vi "Create.vi"(5 "TestFailure In":refnum<class "TestFailure.lvclass">, 8 "error in (no error)":errorcluster, 9 "Failure":errorcluster, 10 "Test":refnum<class "Test.lvclass">) -> (0 "error out":errorcluster, 3 "TestFailure":refnum<class "TestFailure.lvclass">)   [LabVIEW 2019, in "TestFailure.lvclass"]
uses:
  TestFailure.lvclass
  Test/Test.lvclass
  TestFailure.lvclass/TestFailure.ctl
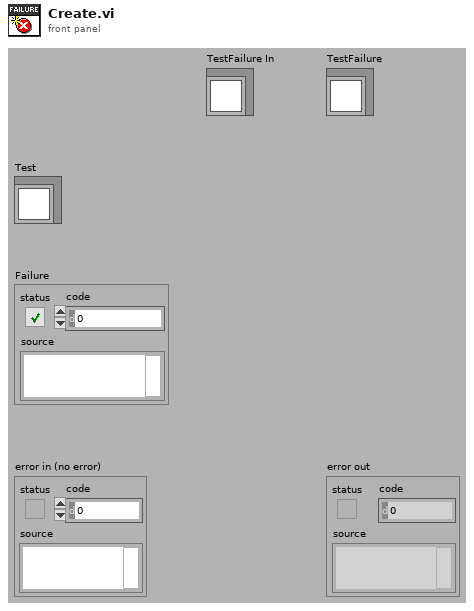
[diagram p1: front panel]
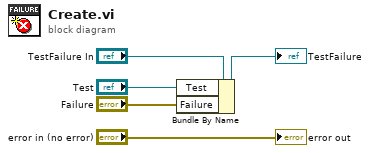
[diagram p0: block diagram]
diagram:
  n1 = Bundle By Name(cluster="TestFailure In", "Test"="Test", "Failure"="Failure") -> (→"TestFailure":refnum<class "TestFailure.lvclass">)
  "error out" <- "error in (no error)"
